vi "Find_VISA.vi"() -> (2 "Com port list":string[](array[string]))   [LabVIEW 2018]
uses:
  <vilib>/Instr/_visa.llb/VISA Find Search Mode.ctl
panel:
  out "返回数":u32
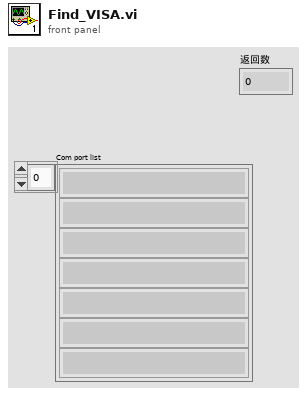
[diagram p1: front panel]
types:
  T1 = typedef "VISA Find Search Mode.ctl" = u32
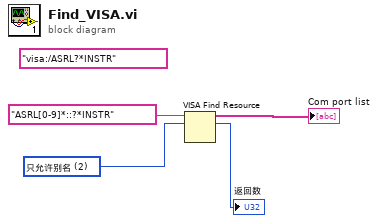
[diagram p0: block diagram]
diagram:
  (unwired) "visa:/ASRL?*INSTR" ("expression (\"?*\")")
  w2 = T1 2 items=["仅允许规范名称"=0, "只允许别名"=2, "包含匹配别名"=3, "包含所有别名"=4] ("Search Mode")
  n1 = VISA Find Resource(10:w2, 11:"ASRL[0-9]*::?*INSTR" ("expression (\"?*\")")) -> (2:→"返回数":u32, 3:→"Com port list":string[])  [unwired: 1 in, 1 out]
